vi "OuputMixer5782_2.vi"(6 "reset":bool, 8 "valid in":bool, 9 "Phase output":fxp<+,64,64>[](array[numeric])=[0.0, 0.0], 11 "Data in":fxp<+/-,16,14>[](array[numeric])=[0.0, 0.0]) -> (0 "valid out":bool)   [LabVIEW 2013]
doc: "Outputs input from channel 0 as I*cos(t)-Q*sin(t) on analog output 0"
uses:
  <vilib>/rvi/eio/common/nirviEmuTemplateMethod_errors.vi
  <vilib>/eio/EIONode/EIONode.xnode
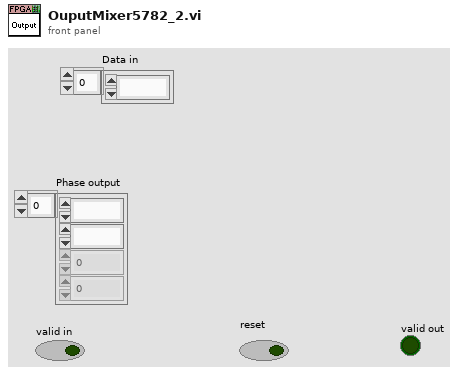
[diagram p1: front panel]
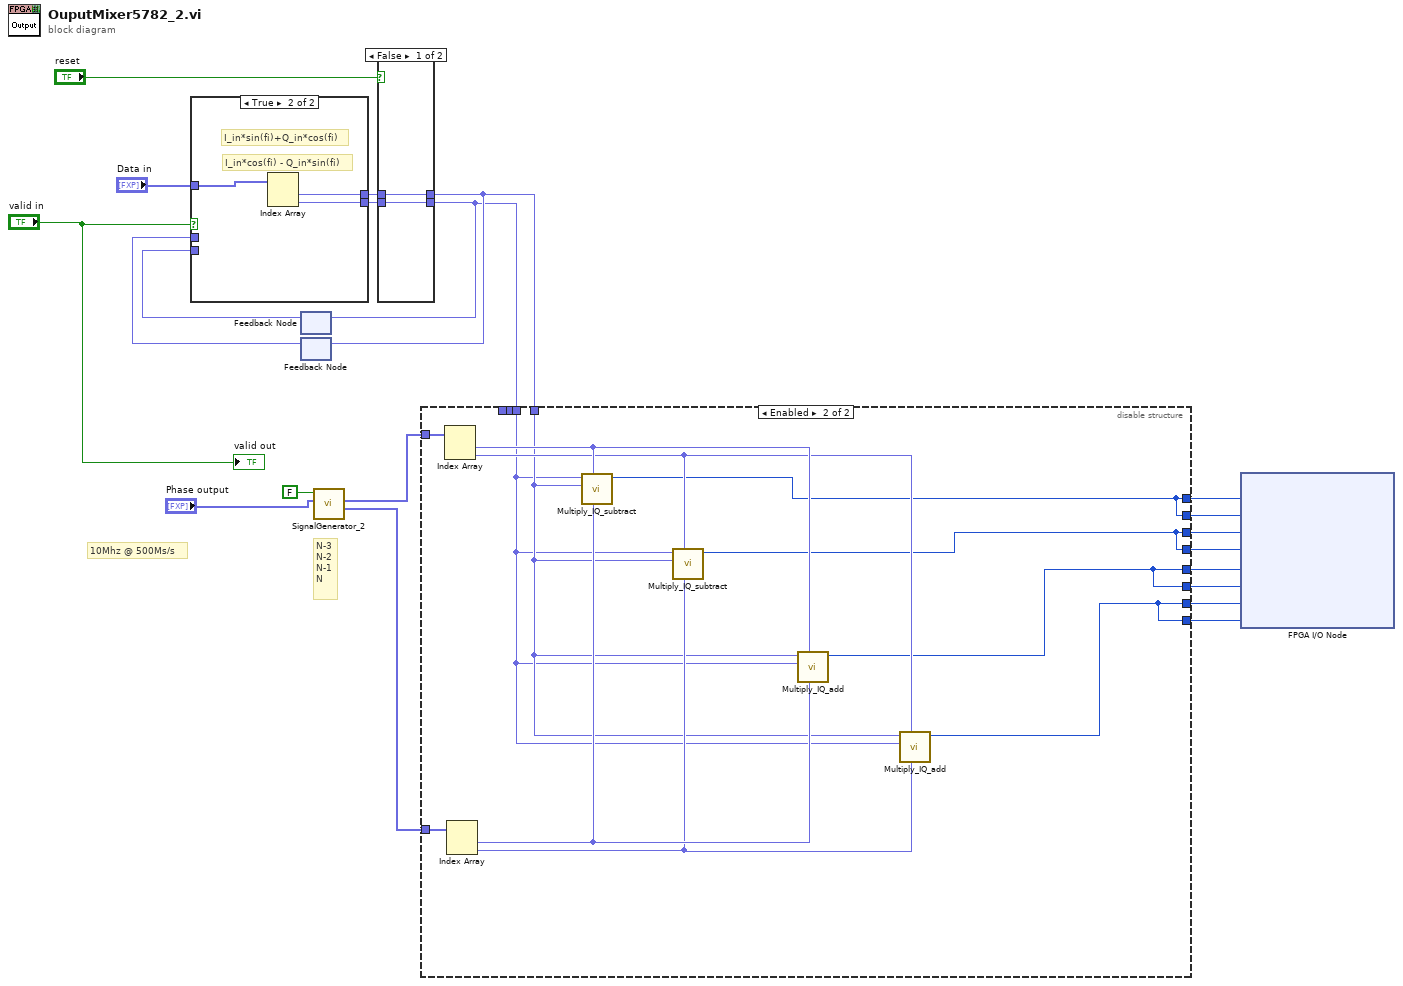
[diagram p0: block diagram]
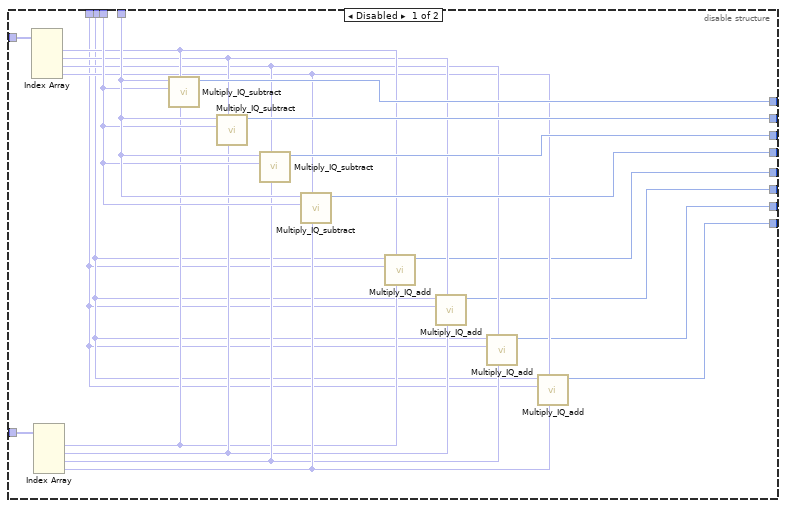
[diagram p2: hidden frame]
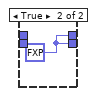
[diagram p3: hidden frame]
diagram:
  # "10Mhz @ 500Ms/s"
  # "N-3\nN-2\nN-1\nN"
  n1 = feedback #1() -> (w14:fxp<+/-,16,14>)  [unwired: 1 in]
  n2 = feedback #2() -> (w13:fxp<+/-,16,14>)  [unwired: 1 in]
  n3 = case shown="True" "valid in" {
    tunnel: "Data in" -> [_ w26]
    tunnel: w14 -> [w22 _]
    tunnel: w13 -> [w23 _]
    tunnel: [w23 w25] -> w12
    tunnel: [w22 w24] -> w11
    frame False {
      # "keep old values"
    }
    frame True {
      # "I_in*cos(fi) - Q_in*sin(fi)"
      # "I_in*sin(fi)+Q_in*cos(fi)"
      n4 = Index Array(array=w26) -> (element #1=w25:fxp<+/-,16,14>, element #2=w24:fxp<+/-,16,14>)  [unwired: 2 in]
    }
  }
  n5 = call "SignalGenerator_2.vi"("Phase"="Phase output", "reset"=FALSE) -> ("Sine out"=w1:fxp<+/-,16,0>[], "Cosine out"=w2:fxp<+/-,16,0>[])  [unwired: 8 in]
  n6 = case shown="False" "reset" {
    tunnel: w12 -> [w27 _]
    tunnel: w11 -> [w28 _]
    tunnel: [w28 w29] -> w9
    tunnel: [w27 w29] -> w10
    frame False {
    }
    frame True {
      w29 = fxp<+/-,16,14> 0.0 ("Q in")
    }
  }
  n7 = feedback-in #1(w9) -> ()
  n8 = feedback-in #2(w10) -> ()
  n9 = disable-structure shown="Enabled" {
    disable-tunnel: w2 -> [w51 w63]
    disable-tunnel: w1 -> [w50 w62]
    disable-tunnel: [w49 w57] -> w21
    disable-tunnel: [w48 w57] -> w20
    disable-tunnel: [w47 w56] -> w19
    disable-tunnel: [w46 w56] -> w18
    disable-tunnel: w10 -> [w45 w53]
    disable-tunnel: w9 -> [w44 w52]
    disable-tunnel: _ -> [w35 _]
    disable-tunnel: _ -> [w34 _]
    disable-tunnel: [w33 w55] -> w8
    disable-tunnel: [w32 w55] -> w7
    disable-tunnel: [w31 w54] -> w6
    disable-tunnel: [w30 w54] -> w5
    frame Disabled {
      n10 = Index Array(array=w51) -> (element #1=w43:fxp<+/-,16,0>, element #2=w42:fxp<+/-,16,0>, element #3=w41:fxp<+/-,16,0>, element #4=w40:fxp<+/-,16,0>)  [unwired: 4 in]
      n11 = Index Array(array=w50) -> (element #1=w36:fxp<+/-,16,0>, element #2=w37:fxp<+/-,16,0>, element #3=w38:fxp<+/-,16,0>, element #4=w39:fxp<+/-,16,0>)  [unwired: 4 in]
      n12 = call "Multiply_IQ_subtract.vi"("Sin"=w36, "Cos"=w43, "Q"=w44, "I"=w45) -> ("Z"=w49:i16)  [unwired: 6 in, 1 out]
      n13 = call "Multiply_IQ_subtract.vi"("Sin"=w37, "Cos"=w42, "Q"=w44, "I"=w45) -> ("Z"=w48:i16)  [unwired: 6 in, 1 out]
      n14 = call "Multiply_IQ_subtract.vi"("Sin"=w38, "Cos"=w41, "Q"=w44, "I"=w45) -> ("Z"=w47:i16)  [unwired: 6 in, 1 out]
      n15 = call "Multiply_IQ_subtract.vi"("Sin"=w39, "Cos"=w40, "Q"=w44, "I"=w45) -> ("Z"=w46:i16)  [unwired: 6 in, 1 out]
      n16 = call "Multiply_IQ_add.vi"("Sin"=w36, "Cos"=w43, "Q"=w34, "I"=w35) -> ("Z"=w33:i16)  [unwired: 6 in, 1 out]
      n17 = call "Multiply_IQ_add.vi"("Sin"=w37, "Cos"=w42, "Q"=w34, "I"=w35) -> ("Z"=w32:i16)  [unwired: 6 in, 1 out]
      n18 = call "Multiply_IQ_add.vi"("Sin"=w38, "Cos"=w41, "Q"=w34, "I"=w35) -> ("Z"=w31:i16)  [unwired: 6 in, 1 out]
      n19 = call "Multiply_IQ_add.vi"("Sin"=w39, "Cos"=w40, "Q"=w34, "I"=w35) -> ("Z"=w30:i16)  [unwired: 6 in, 1 out]
    }
    frame Enabled {
      n20 = Index Array(array=w63) -> (element #1=w61:fxp<+/-,16,0>, element #2=w59:fxp<+/-,16,0>)  [unwired: 2 in]
      n21 = Index Array(array=w62) -> (element #1=w60:fxp<+/-,16,0>, element #2=w58:fxp<+/-,16,0>)  [unwired: 2 in]
      n22 = call "Multiply_IQ_subtract.vi"("Sin"=w60, "Cos"=w61, "Q"=w53, "I"=w52) -> ("Z"=w57:i16)  [unwired: 6 in, 1 out]
      n23 = call "Multiply_IQ_subtract.vi"("Sin"=w58, "Cos"=w59, "Q"=w53, "I"=w52) -> ("Z"=w56:i16)  [unwired: 6 in, 1 out]
      n24 = call "Multiply_IQ_add.vi"("Sin"=w60, "Cos"=w61, "Q"=w52, "I"=w53) -> ("Z"=w55:i16)  [unwired: 6 in, 1 out]
      n25 = call "Multiply_IQ_add.vi"("Sin"=w58, "Cos"=w59, "Q"=w52, "I"=w53) -> ("Z"=w54:i16)  [unwired: 6 in, 1 out]
    }
  }
  n26 = xnode "FPGA I/O Node"("IO Module\\AO 0 N-3"=w21, "IO Module\\AO 0 N-2"=w20, "IO Module\\AO 0 N-1"=w19, "IO Module\\AO 0 N"=w18, "IO Module\\AO 1 N-3"=w8, "IO Module\\AO 1 N-2"=w7, "IO Module\\AO 1 N-1"=w6, "IO Module\\AO 1 N"=w5) -> ()  [unwired: 8 in, 8 out]
  "valid out" <- "valid in"
